vi "BuscaPlaca_USB_NI.vi"(8 "error in (no error)":errorcluster) -> (0 "error out":errorcluster, 2 "PlacasRing":cluster{"String":string, "Value":u16}[](array[cluster]), 3 "HardwareConfiguration":T2(array[cluster]))   [LabVIEW 2019]
uses:
  <vilib>/Utility/miscctls.llb/LVStringsAndValuesArrayTypeDef_U16.ctl
  <resource>/objmgr/daqmx.rc
panel:
  in  "IncludeSimulated":bool=TRUE
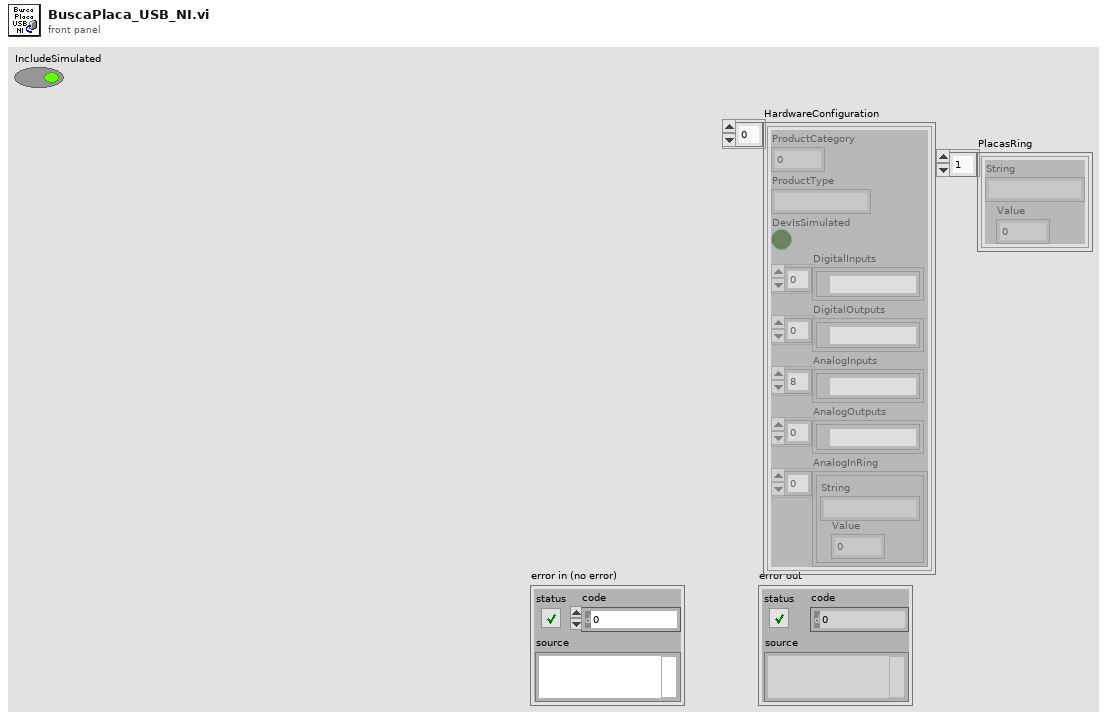
[diagram p1: front panel]
types:
  T1 = typedef "LVStringsAndValuesArrayTypeDef_U16.ctl" = cluster{"String":string, "Value":u16}[]
  T2 = cluster{"ProductCategory":i32, "ProductType":string, "DevIsSimulated":bool, "DigitalInputs":tag[], "DigitalOutputs":tag[], "AnalogInputs":tag[], "AnalogOutputs":tag[], "AnalogInRing":T1}[]
  T3 = cluster{"ProductCategory":i32, "ProductType":string, "DevIsSimulated":bool, "DigitalInputs":tag[], "DigitalOutputs":tag[], "AnalogInputs":tag[], "AnalogOutputs":tag[], "AnalogInRing":T1}
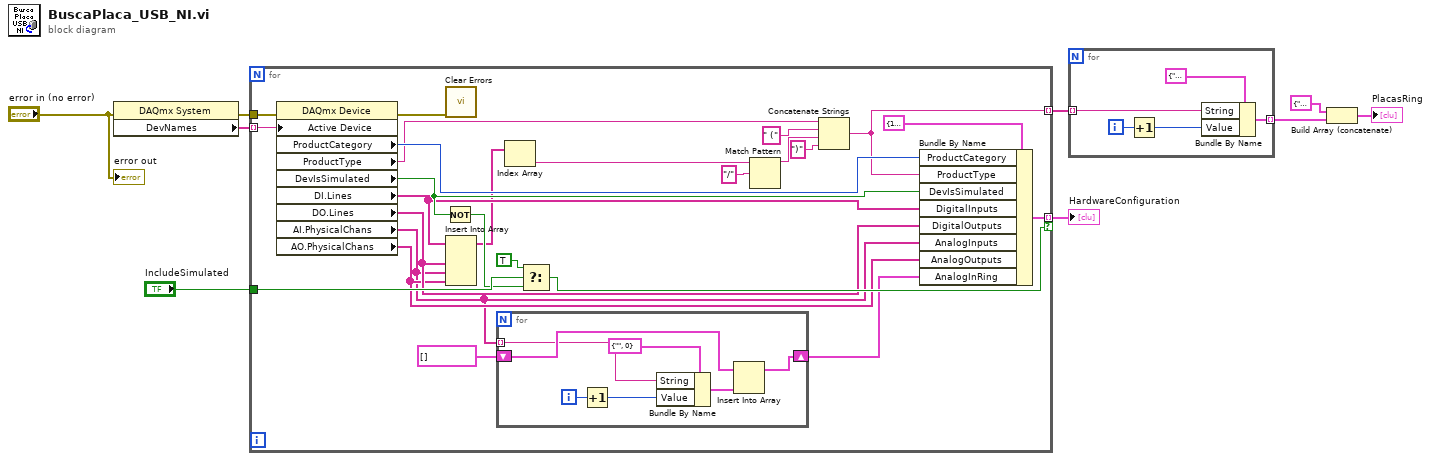
[diagram p0: block diagram]
diagram:
  n1 = property class="DAQmx System"(error in="error in (no error)") -> (error out=w8:errorcluster, "DevNames"=w9:tag[])  [unwired: 1 in, 1 out]
  n2 = for {
    tunnel: w9 -> [w34] mode=indexing
    tunnel: [w32] -> w5 mode=indexing if=w24
    tunnel: w8 -> [w30]
    tunnel: "IncludeSimulated" -> [w27]
    tunnel: [w10] -> w4 mode=indexing
    n3 = property class="DAQmx Device"(error in=w30, "Active Device"=w34) -> (error out=w29:errorcluster, "ProductCategory"=w31:i32, "ProductType"=w17:string, "DevIsSimulated"=w28:bool, "DI.Lines"=w23:tag[], "DO.Lines"=w22:tag[], "AI.PhysicalChans"=w13:tag[], "AO.PhysicalChans"=w21:tag[])  [unwired: 1 in, 1 out]
    n4 = Not(x=w28) -> (.not. x?=w26:bool)
    n5 = call <vilib>:"Clear Errors.vi"("error in (no error)"=w29) -> ()  [unwired: 5 in, 2 out]
    n6 = Insert Into Array(array=w23, new element #1=w22, new element #2=w13, new element #3=w21) -> (w20:tag[])  [unwired: 1 in]
    n7 = for {
      tunnel: w13 -> [w39] mode=indexing
      shift-right: [w36] -> w11
      shift-left: T1 [] ("Strings And Values []") -> [w41]
      i -> [w38]
      n8 = Increment(x=w38) -> (x+1=w35:i32)
      n9 = Bundle By Name(cluster=cluster{"String":string, "Value":u16} {"String"="", "Value"=0}, "String"=w39, "Value"=w35) -> (w37:cluster{"String":string, "Value":u16})
      n10 = Insert Into Array(array=w41, new element=w37) -> (w36:T1)  [unwired: 1 in]
    }
    n11 = Index Array(array=w20) -> (element=w19:tag)  [unwired: 1 in]
    n12 = Select(t=TRUE, s=w27, f=w26) -> (s? t:f=w24:bool)
    n13 = Match Pattern(string=w19, regular expression="/") -> (before substring=w16:string)  [unwired: 1 in, 3 out]
    n14 = Concatenate Strings(w17, " (" ("string"), w16, ")" ("string")) -> (w10:string)
    n15 = Bundle By Name(cluster=T3 {"ProductCategory"=14643, "ProductType"="", "DevIsSimulated"=FALSE, "DigitalInputs"=[], "DigitalOutputs"=[], "AnalogInputs"=[], "AnalogOutputs"=[], "AnalogInRing"=[]}, "ProductCategory"=w31, "ProductType"=w10, "DevIsSimulated"=w28, "DigitalInputs"=w23, "DigitalOutputs"=w22, "AnalogInputs"=w13, "AnalogOutputs"=w21, "AnalogInRing"=w11) -> (w32:T3)
  }
  "HardwareConfiguration" <- w5
  n16 = for {
    tunnel: w4 -> [w45] mode=indexing
    tunnel: [w42] -> w3 mode=indexing
    i -> [w44]
    n17 = Increment(x=w44) -> (x+1=w43:i32)
    n18 = Bundle By Name(cluster=cluster{"String":string, "Value":u16} {"String"="None", "Value"=0}, "String"=w45, "Value"=w43) -> (w42:cluster{"String":string, "Value":u16})
  }
  n19 = Build Array (concatenate)(cluster{"String":string, "Value":u16} {"String"="None", "Value"=0}, w3) -> (→"PlacasRing":cluster{"String":string, "Value":u16}[])
  "error out" <- "error in (no error)"
